vi "Board PSU server.vi"() -> ()   [LabVIEW 2025]
uses:
  <userlib>/_OpenG.lib/comparison/comparison.llb/Boolean Changed__ogtk.vi
  <userlib>/_OpenG.lib/comparison/comparison.llb/DBL Changed__ogtk.vi
  Program Files/National Instruments/LabVIEW 2024/instr.lib/CPX200DP/CPX200DP.lvlib
  <userlib>/_OpenG.lib/comparison/comparison.llb/openg_comparison__ogtk.lvlib
panel:
  in  "Current Limit (150mA)":dbl=0.15 format="%.2g"
  out "PSU_Monitor":waveform(dbl)[](array[waveform])=[{"t0"=timestamp(3820238929.2708097 s since 1904-01-01), "dt"=1.0, "Y"=[-0.003], "attributes"=variant("NI_ChannelName"=variant(string "Board_Voltage_0"))}, {"t0"=timestamp(3820238929.279827 s since 1904-01-01), "dt"=1.0, "Y"=[-0.01], "attributes"=variant("NI_ChannelName"=variant(string "Board_Voltage_0"))}]
  out "PSU_Voltages":waveform(dbl)[](array[waveform])=[{"t0"=timestamp(3820238929.2708097 s since 1904-01-01), "dt"=1.0, "Y"=[-0.003], "attributes"=variant("NI_ChannelName"=variant(string "Board_Voltage_0"))}, {"t0"=timestamp(3820238929.279827 s since 1904-01-01), "dt"=1.0, "Y"=[-0.01], "attributes"=variant("NI_ChannelName"=variant(string "Board_Voltage_0"))}]
  out "PSU_Currents":waveform(dbl)[](array[waveform])=[{"t0"=timestamp(3820238929.2708097 s since 1904-01-01), "dt"=1.0, "Y"=[0.003], "attributes"=variant("NI_ChannelName"=variant(string "Board_Current_0"))}, {"t0"=timestamp(3820238929.279827 s since 1904-01-01), "dt"=1.0, "Y"=[0.001], "attributes"=variant("NI_ChannelName"=variant(string "Board_Current_0"))}]
  in  "Board PSU \nVISA name":refnum<visa-resource-name>="CPX200PSU"
  in  "Cadence (ms)":i64=100 min=1 max=1000
  out "I&V (Graph)":dynamicdata(graph)=[{"t0"=timestamp(3820238929.2708097 s since 1904-01-01), "dt"=1.0, "Y"=[-0.003], "attributes"=variant("NI_ChannelName"=variant(string "Board_Voltage_0"))}, {"t0"=timestamp(3820238929.279827 s since 1904-01-01), "dt"=1.0, "Y"=[-0.01], "attributes"=variant("NI_ChannelName"=variant(string "Board_Voltage_0"))}, {"t0"=timestamp(3820238929.2708097 s since 1904-01-01), "dt"=1.0, "Y"=[0.003], "attributes"=variant("NI_ChannelName"=variant(string "Board_Current_0"))}, {"t0"=timestamp(3820238929.279827 s since 1904-01-01), "dt"=1.0, "Y"=[0.001], "attributes"=variant("NI_ChannelName"=variant(string "Board_Current_0"))}]
  in  "stop":bool
  in  "Enable Output (T: Enable)":bool
  in  "Set Voltage":dbl=12.0 min=0.0 max=15.0 step=1.0 format="%.2f"
  in  "OCP Current (A)":dbl=0.15
  in  "OVP Voltage (V)":dbl=15.0
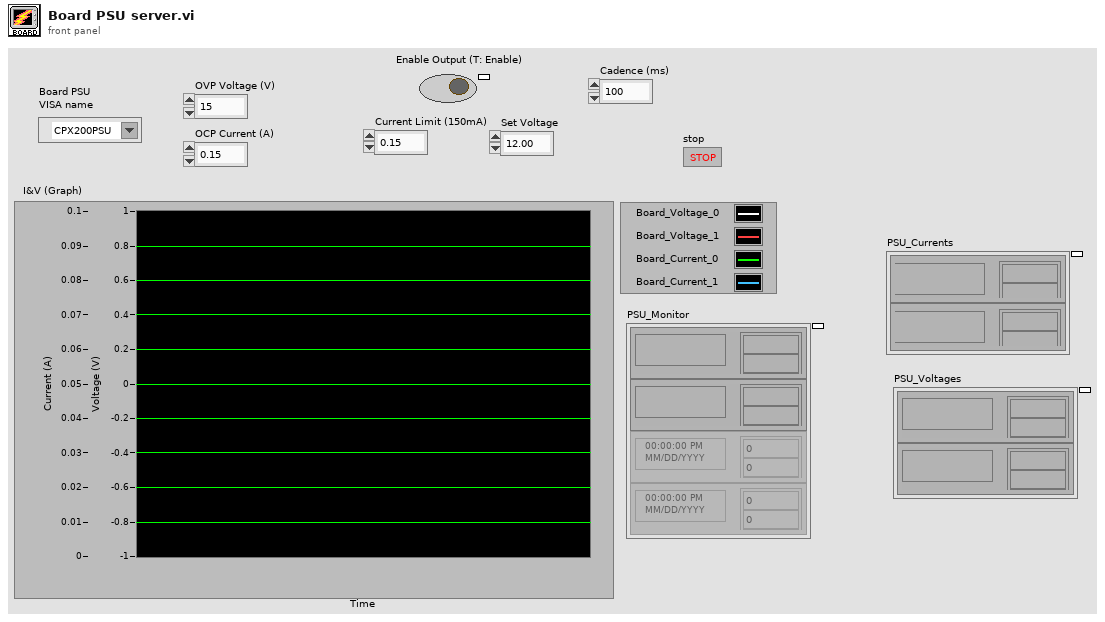
[diagram p1: front panel]
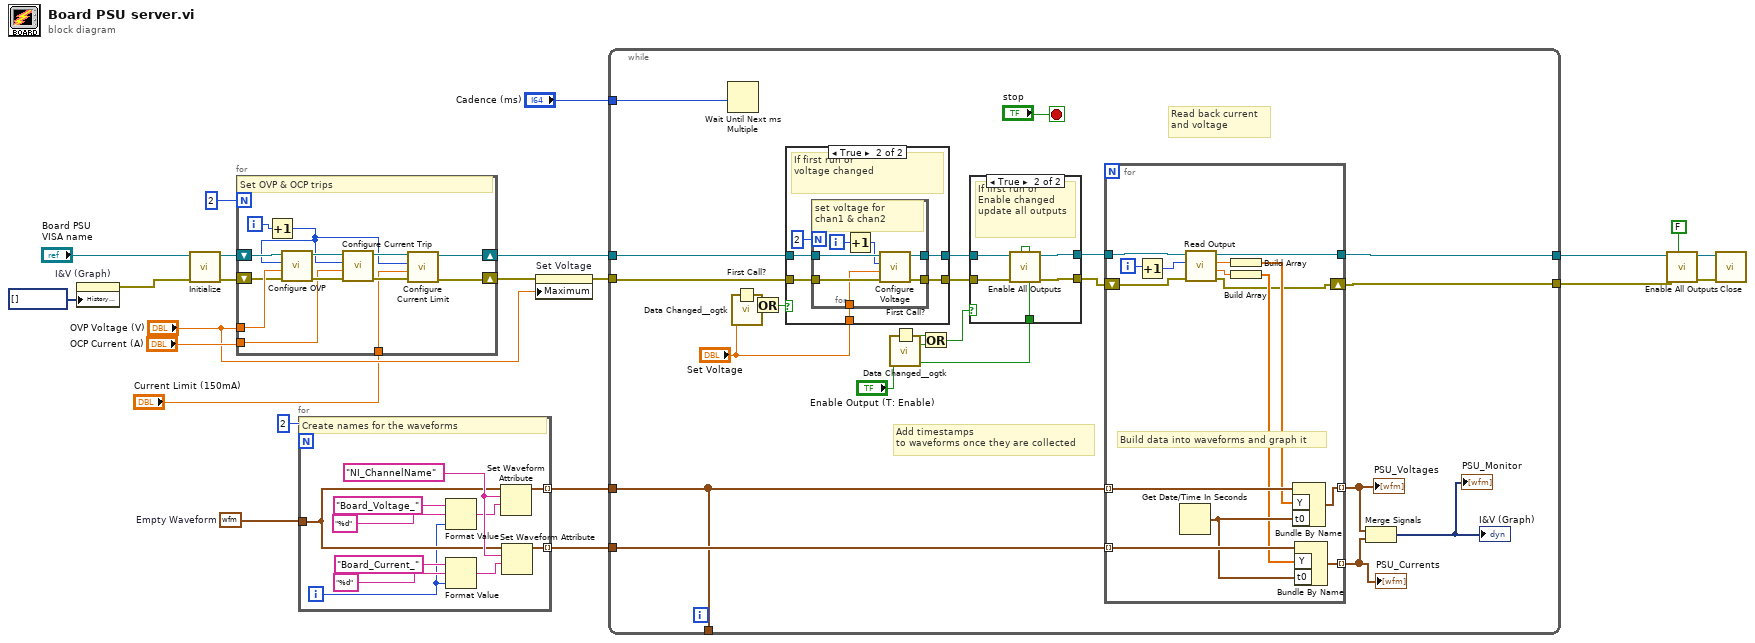
[diagram p0: block diagram]
diagram:
  w17 = waveform(dbl) {"t0"=timestamp(0 s since 1904-01-01), "dt"=1.0, "Y"=[]}  # Empty Waveform
  n1 = property on="I&V (Graph)" class="WFChart (strict)"("History Data"=dynamicdata[] []) -> (error out=w8:errorcluster)  [unwired: 2 in, 1 out]
  n2 = call "Initialize.vi"("error in (no error)"=w8, "VISA resource name"="Board PSU \nVISA name") -> ("error out"=w10:errorcluster, "VISA resource name out"=w15:refnum<visa-resource-name>)  [unwired: 8 in]
  n3 = for {
    N: 2 -> [_]
    tunnel: "OCP Current (A)" -> [w33]
    tunnel: "OVP Voltage (V)" -> [w32]
    shift-right: [w26] -> w3
    shift-left: w15 -> [w31]
    shift-right: [w25] -> w4
    shift-left: w10 -> [w30]
    tunnel: "Current Limit (150mA)" -> [w23]
    i -> [w29]
    # "Set OVP & OCP trips"
    n4 = Increment(x=w29) -> (x+1=w24:i32)
    n5 = call "Configure OVP.vi"("error in (no error)"=w30, "Voltage Limit (0.0 V)"=w32, "Channel (1: Channel 1)"=w24, "VISA resource name"=w31) -> ("error out"=w35:errorcluster, "VISA resource name out"=w34:refnum<visa-resource-name>)  [unwired: 6 in]
    n6 = call "Configure Current Trip.vi"("error in (no error)"=w35, "Current Limit (0.0 A)"=w33, "Channel (1: Channel 1)"=w24, "VISA resource name"=w34) -> ("error out"=w27:errorcluster, "VISA resource name out"=w28:refnum<visa-resource-name>)  [unwired: 6 in]
    n7 = call "Configure Current Limit.vi"("error in (no error)"=w27, "Current Limit (0.0 A)"=w23, "Channel (1: Channel 1)"=w24, "VISA resource name"=w28) -> ("error out"=w25:errorcluster, "VISA resource name out"=w26:refnum<visa-resource-name>)  [unwired: 6 in]
  }
  n8 = for {
    N: 2 -> [_]
    tunnel: [w46] -> w12 mode=indexing
    tunnel: w17 -> [w44]
    tunnel: [w43] -> w11 mode=indexing
    i -> [w36]
    w45 = "NI_ChannelName" ("name")
    # "Create names for the waveforms"
    n9 = Format Value(string ("")="Board_Voltage_", format string="%d", value (0)=w36) -> (output string=w41:string)
    n10 = Format Value(string ("")="Board_Current_", format string="%d", value (0)=w36) -> (output string=w39:string)
    n11 = Set Waveform Attribute(5:w41, 6:w45, 7:w44) -> (3:w46:waveform(dbl))  [unwired: 1 in, 2 out]
    n12 = Set Waveform Attribute(5:w39, 6:w45, 7:w44) -> (3:w43:waveform(dbl))  [unwired: 1 in, 2 out]
  }
  n13 = property on="Set Voltage" class="DigNum (strict)"(error in=w4, "Maximum"="OVP Voltage (V)") -> (error out=w2:errorcluster)  [unwired: 1 in, 1 out]
  n14 = while {
    tunnel: w2 -> [w69]
    tunnel: w12 -> [w49]
    tunnel: w11 -> [w66]
    tunnel: [w65] -> w7
    tunnel: [w60] -> w6
    tunnel: w3 -> [w61]
    tunnel: [w49] -> _
    tunnel: "Cadence (ms)" -> [w47]
    stop <- "stop" stop-if-true
    # "Add timestamps\nto waveforms once they are collected"
    # "Read back current \nand voltage"
    n15 = Wait Until Next ms Multiple(millisecond multiple=w47) -> ()  [unwired: 1 out]
    n16 = First Call?() -> (First Call?: T/F=w57:bool)
    n17 = call-poly <userlib>:"Data Changed__ogtk.vi"("DBL"="Set Voltage") -> ("Changed"=w58:bool)
    n18 = Or(x=w57, y=w58) -> (x .or. y?=w59:bool)
    n19 = case shown="True" w59 {
      tunnel: w61 -> [w78 w84]
      tunnel: w69 -> [w77 w83]
      tunnel: "Set Voltage" -> [_ w82]
      tunnel: [w78 w81] -> w51
      tunnel: [w77 w80] -> w52
      frame False {
      }
      frame True {
        # "If first run or\nvoltage changed"
        n20 = for {
          N: 2 -> [_]
          tunnel: w84 -> [w90]
          tunnel: w83 -> [w91]
          tunnel: [w87] -> w81
          tunnel: [w86] -> w80
          tunnel: w82 -> [w85]
          i -> [w89]
          # "set voltage for \nchan1 & chan2"
          n21 = Increment(x=w89) -> (x+1=w88:i32)
          n22 = call "Configure Voltage.vi"("error in (no error)"=w91, "Voltage (0.0 V)"=w85, "Channel (1: Channel 1)"=w88, "VISA resource name"=w90) -> ("error out"=w86:errorcluster, "VISA resource name out"=w87:refnum<visa-resource-name>)  [unwired: 6 in]
        }
      }
    }
    n23 = call-poly <userlib>:"Data Changed__ogtk.vi"("Boolean"="Enable Output (T: Enable)") -> ("Changed"=w54:bool)
    n24 = First Call?() -> (First Call?: T/F=w55:bool)
    n25 = Or(x=w55, y=w54) -> (x .or. y?=w53:bool)
    n26 = case shown="True" w53 {
      tunnel: w52 -> [w70 w76]
      tunnel: w51 -> [w71 w75]
      tunnel: "Enable Output (T: Enable)" -> [_ w74]
      tunnel: [w71 w73] -> w68
      tunnel: [w70 w72] -> w67
      frame False {
      }
      frame True {
        # "If first run or\nEnable changed\nupdate all outputs"
        n27 = call "Enable All Outputs.vi"("Enable Output (T: Enable)"=w74, "error in (no error)"=w76, "VISA resource name"=w75) -> ("error out"=w72:errorcluster, "VISA resource name out"=w73:refnum<visa-resource-name>)  [unwired: 7 in]
      }
    }
    n28 = for {
      tunnel: w68 -> [w105]
      tunnel: w49 -> [w102] mode=indexing
      tunnel: w66 -> [w101] mode=indexing
      tunnel: [w103] -> w65
      tunnel: [w97] -> w62 mode=indexing
      tunnel: [w96] -> w63 mode=indexing
      shift-right: [w95] -> w60
      shift-left: w67 -> [w104]
      i -> [w106]
      # "Build data into waveforms and graph it"
      n29 = Increment(x=w106) -> (x+1=w94:i32)
      n30 = Get Date/Time In Seconds() -> (seconds since 1Jan1904=w100:timestamp)
      n31 = call "Read Output.vi"("error in (no error)"=w104, "Channel (1: Channel 1)"=w94, "VISA resource name"=w105) -> ("error out"=w95:errorcluster, "Actual Current Level (A)"=w92:dbl, "Actual Voltage Level (V)"=w93:dbl, "VISA resource name out"=w103:refnum<visa-resource-name>)  [unwired: 5 in]
      n32 = Build Array(w93) -> (w98:dbl[])
      n33 = Build Array(w92) -> (w99:dbl[])
      n34 = Bundle By Name(cluster=w102, "Y"=w98, "t0"=w100) -> (w96:waveform(dbl))
      n35 = Bundle By Name(cluster=w101, "Y"=w99, "t0"=w100) -> (w97:waveform(dbl))
    }
    "PSU_Currents" <- w62
    "PSU_Voltages" <- w63
    n36 = Merge Signals(w63, w62) -> (→"I&V (Graph)" →"PSU_Monitor":dynamicdata)
  }
  n37 = call "Enable All Outputs.vi"("Enable Output (T: Enable)"=FALSE, "error in (no error)"=w6, "VISA resource name"=w7) -> ("error out"=w20:errorcluster, "VISA resource name out"=w19:refnum<visa-resource-name>)  [unwired: 7 in]
  n38 = call "Close.vi"("error in (no error)"=w20, "VISA resource name"=w19) -> ()  [unwired: 9 in, 1 out]
